vi "AutoScale.vi"(5 "ScaleOrdinate 2":T1(ring)=enum."Проценты" caption="Ось ординат", 7 "Type_signal":T2(ring), 11 "UNDT_Gain":dbl) -> (1 "Minor":dbl, 2 "Min":dbl, 3 "Max":dbl)   [LabVIEW 2017]
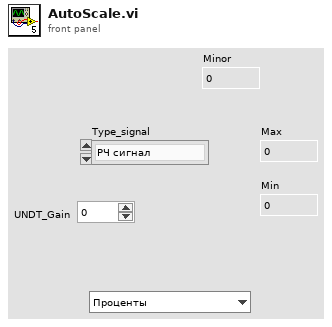
[diagram p1: front panel]
types:
  T1 = enum16{"Отсчеты АЦП (±32767)", "Проценты", "Вольты", "дБмкВ (отн. 1 мкВ)", "Отсчеты АЦП (±1)"}
  T2 = enum16{"РЧ сигнал", "Детект. полное", "Положит.", "Отрицат."}
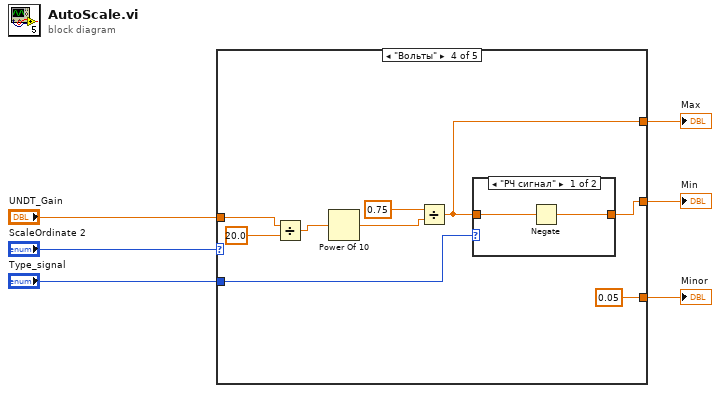
[diagram p0: block diagram]
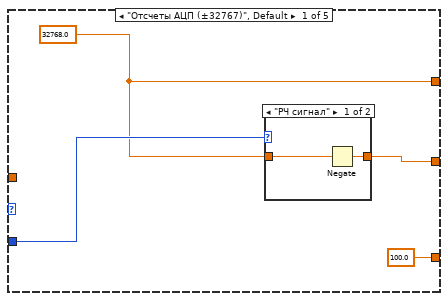
[diagram p2: hidden frame]
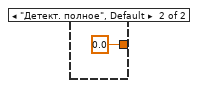
[diagram p3: hidden frame]
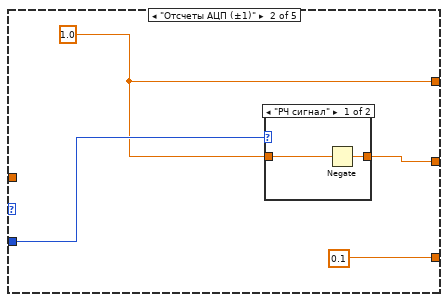
[diagram p4: hidden frame]
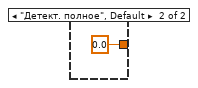
[diagram p5: hidden frame]
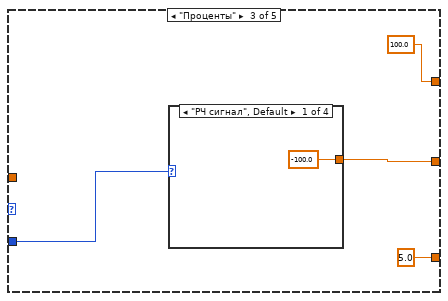
[diagram p6: hidden frame]
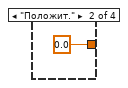
[diagram p7: hidden frame]
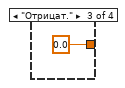
[diagram p8: hidden frame]
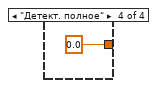
[diagram p9: hidden frame]
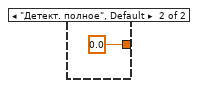
[diagram p10: hidden frame]
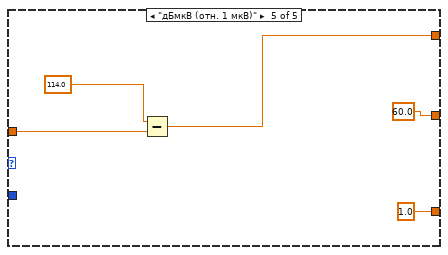
[diagram p11: hidden frame]
diagram:
  n1 = case shown="\"Вольты\"" "ScaleOrdinate 2" {
    tunnel: [w8 w15 100.0 w32 w42] -> w6
    tunnel: [w10 w17 w22 w31 60.0] -> w5
    tunnel: "UNDT_Gain" -> [_ _ _ w37 w43]
    tunnel: "Type_signal" -> [w9 w16 w23 w30 _]
    tunnel: [100.0 0.1 5.0 0.05 1.0] -> w1
    frame "Отсчеты АЦП (±32767)", Default {
      w8 = 32768.0
      n2 = case shown="\"РЧ сигнал\"" w9 {
        tunnel: w8 -> [w12 _]
        tunnel: [w11 0.0] -> w10
        frame "РЧ сигнал" {
          n3 = Negate(x=w12) -> (-x=w11:dbl)
        }
        frame "Детект. полное", Default {
        }
      }
    }
    frame "Отсчеты АЦП (±1)" {
      w15 = 1.0
      n4 = case shown="\"РЧ сигнал\"" w16 {
        tunnel: w15 -> [w19 _]
        tunnel: [w18 0.0] -> w17
        frame "РЧ сигнал" {
          n5 = Negate(x=w19) -> (-x=w18:dbl)
        }
        frame "Детект. полное", Default {
        }
      }
    }
    frame "Проценты" {
      n6 = case shown="\"РЧ сигнал\", Default" w23 {
        tunnel: [-100.0 0.0 0.0 0.0] -> w22
        frame "РЧ сигнал", Default {
        }
        frame "Положит." {
        }
        frame "Отрицат." {
        }
        frame "Детект. полное" {
        }
      }
    }
    frame "Вольты" {
      n7 = Divide(x=w37, y=20.0) -> (x/y=w35:dbl)
      n8 = Power Of 10(x=w35) -> (10^x=w33:dbl)
      n9 = Divide(x=0.75, y=w33) -> (x/y=w32:dbl)
      n10 = case shown="\"РЧ сигнал\"" w30 {
        tunnel: w32 -> [w39 _]
        tunnel: [w38 0.0] -> w31
        frame "РЧ сигнал" {
          n11 = Negate(x=w39) -> (-x=w38:dbl)
        }
        frame "Детект. полное", Default {
        }
      }
    }
    frame "дБмкВ (отн. 1 мкВ)" {
      n12 = Subtract(x=114.0, y=w43) -> (x-y=w42:dbl)
    }
  }
  "Min" <- w5
  "Max" <- w6
  "Minor" <- w1
